vi "Pre-Build Custom Action.vi"(10 "Variant":variant) -> (0 "error out":errorcluster)   [LabVIEW 2021]
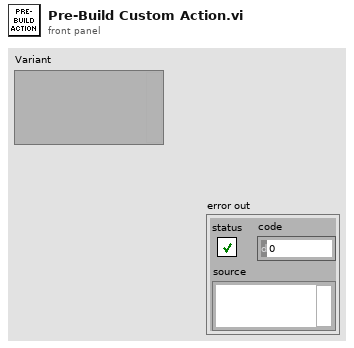
[diagram p1: front panel]
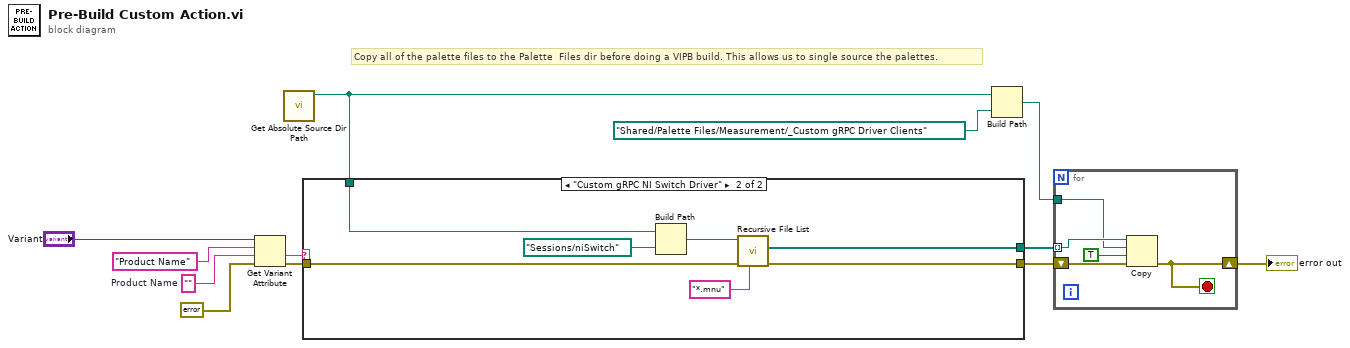
[diagram p0: block diagram]
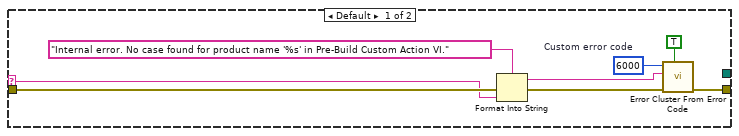
[diagram p2: hidden frame]
diagram:
  w11 = ""  # Product Name
  # "Copy all of the palette files to the Palette  Files dir before doing a VIPB build. This allows us to single source the palettes."
  n1 = Get Variant Attribute(Variant="Variant", name="Product Name", default value (empty Variant)=w11, error in=errorcluster {"status"=FALSE, "code"=0, "source"=""}) -> (value=w2:string, error out=w5:errorcluster)  [unwired: 2 out]
  n2 = call "Get Absolute Source Dir Path.vi"() -> ("source dir"=w1:path)  [unwired: 10 in, 1 out]
  n3 = case shown="\"Custom gRPC NI Switch Driver\"" w2 {
    selector: w2 -> [w13 _]
    tunnel: [_ w26] -> w9
    tunnel: [w15 w25] -> w8
    tunnel: w5 -> [w14 w24]
    tunnel: w1 -> [_ w21]
    frame Default {
      w19 = 6000  # Custom error code
      n4 = Format Into String(format string="Internal error. No case found for product name '%s' in Pre-Build Custom Action VI.", error in=w14, w13) -> (resulting string=w16:string, error out=w20:errorcluster)  [unwired: 1 in]
      n5 = call <vilib>:"Error Cluster From Error Code.vi"("show call chain? (False)"=TRUE, "error in (no error)"=w20, "error message (\"\")"=w16, "error code (0)"=w19) -> ("error out"=w15:errorcluster)  [unwired: 5 in]
    }
    frame "Custom gRPC NI Switch Driver" {
      n6 = Build Path(base path=w21, name or relative path=path "Sessions/niSwitch") -> (appended path=w22:path)
      n7 = call <vilib>:"Recursive File List.vi"("pattern"="*.mnu", "error in (no error)"=w24, "Folder Path"=w22) -> ("error out"=w25:errorcluster, "All Files in Dir"=w26:path[])  [unwired: 4 in, 3 out]
    }
  }
  n8 = Build Path(base path=w1, name or relative path=path "Shared/Palette Files/Measurement/_Custom gRPC Driver Clients") -> (appended path=w6:path)
  n9 = for {
    tunnel: w9 -> [w30] mode=indexing
    tunnel: w6 -> [w29]
    shift-right: [w28] -> w4
    shift-left: w8 -> [w32]
    stop <- w28 stop-if-true
    n10 = Copy(8:w32, 9:TRUE ("overwrite (F)"), 10:w29, 11:w30) -> (0:w28:errorcluster)  [unwired: 1 in, 2 out]
  }
  "error out" <- w4
